vi "WaitForBusInputTrigger.vi"(8 "Error In":errorcluster, 10 "Timeout (ms)":u32, 11 "Keithley 2602 In":refnum<visa-resource-name>) -> (0 "Error Out":errorcluster, 3 "Keithley 2602 Out":refnum<visa-resource-name>)   [LabVIEW 2012]
uses:
  HardwareAbortGlobalAction.ctl
  driver/Keithley-2602.lvlib
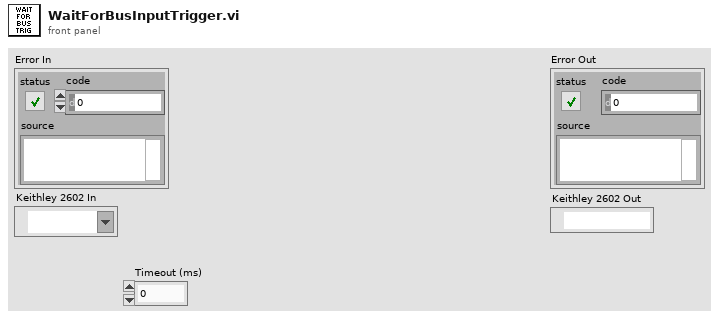
[diagram p1: front panel]
types:
  T1 = typedef "HardwareAbortGlobalAction.ctl" = enum16{"Set", "Get"}
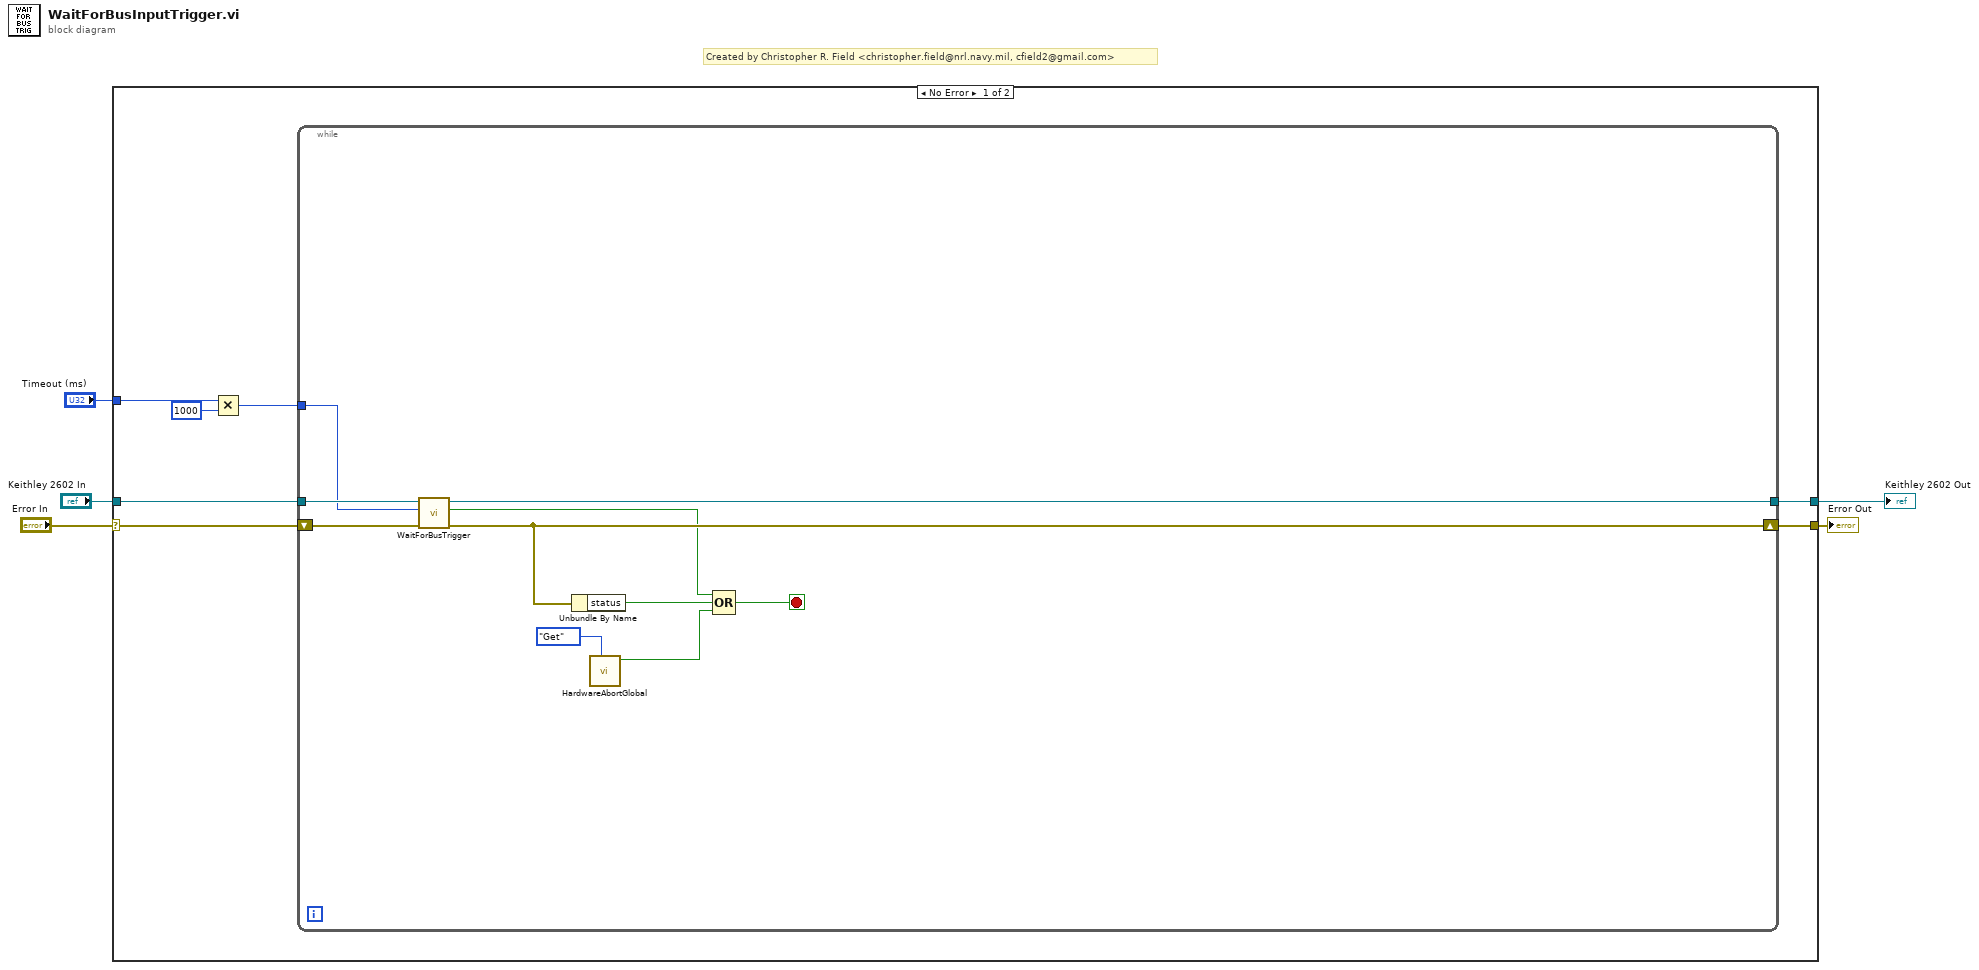
[diagram p0: block diagram]
diagram:
  # "Created by Christopher R. Field <christopher.field@nrl.navy.mil, cfield2@gmail.com>"
  n1 = case shown="No Error" "Error In" {
    selector: "Error In" -> [w12 w23]
    tunnel: [w11 w23] -> w4
    tunnel: "Keithley 2602 In" -> [w10 w24]
    tunnel: [w9 w24] -> w2
    tunnel: "Timeout (ms)" -> [w8 _]
    frame No Error {
      n2 = Multiply(x=w8, y=u32 1000) -> (x*y=w6:u32)
      n3 = while {
        shift-right: [w21] -> w11
        shift-left: w12 -> [w19]
        tunnel: w10 -> [w20]
        tunnel: [w22] -> w9
        tunnel: w6 -> [w18]
        stop <- w15 stop-if-true
        n4 = call "WaitForBusTrigger.vi"("Error In"=w19, "Timeout (sec)"=w18, "Keithley 2602 In"=w20) -> ("Error Out"=w21:errorcluster, "Trigger Detected?"=w17:bool, "Keithley 2602 Out"=w22:refnum<visa-resource-name>)  [unwired: 6 in]
        n5 = Unbundle By Name(w21) -> ("status"=w16:bool)
        n6 = call "HardwareAbortGlobal.vi"("Action"=HardwareAbortGlobalAction."Get") -> ("Value Out"=w13:bool)  [unwired: 10 in]
        n7 = Compound Arithmetic op=OR(w17, w16, w13) -> (w15:bool)
      }
    }
    frame Error {
    }
  }
  "Error Out" <- w4
  "Keithley 2602 Out" <- w2
